vi "sub_SDR_siso_AWGN_channel.vi"(10 "Channel conf":T1, 11 "Shaped symbols":cdb[](array[numeric])) -> (3 "Array":cdb[](array[numeric]))   [LabVIEW 2012]
uses:
  <vilib>/Analysis/NI_AALBase.lvlib
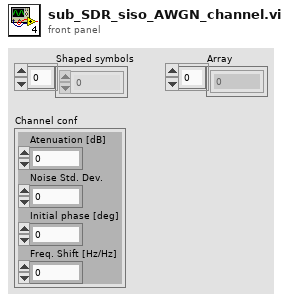
[diagram p1: front panel]
types:
  T1 = cluster{"Atenuation [dB]":dbl, "Noise Std. Dev.":dbl, "Initial phase [deg]":dbl, "Freq. Shift [Hz/Hz]":dbl}
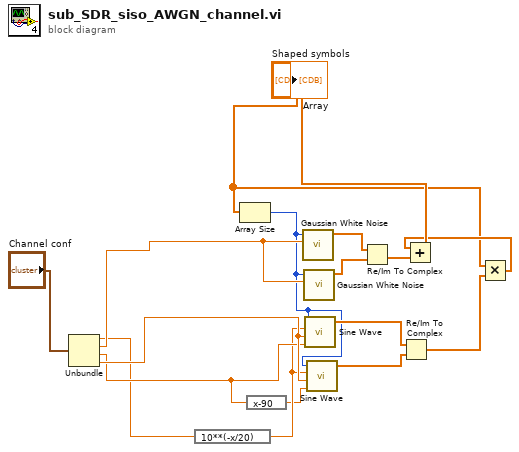
[diagram p0: block diagram]
diagram:
  n1 = Unbundle("Channel conf") -> ("Atenuation [dB]"=w14:dbl, "Noise Std. Dev."=w15:dbl, "Initial phase [deg]"=w16:dbl, "Freq. Shift [Hz/Hz]"=w17:dbl)
  n2 = expression code="10**(-x/20)"(w14) -> (w5:dbl)
  n3 = Array Size(array="Shaped symbols") -> (size(s)=w6:i32)
  n4 = expression code="x-90"(w16) -> (w4:dbl)
  n5 = call <vilib>:"Gaussian White Noise.vi"("standard deviation"=w15, "samples"=w6) -> ("Gaussian noise pattern"=w1:dbl[])  [unwired: 8 in, 1 out]
  n6 = call <vilib>:"Gaussian White Noise.vi"("standard deviation"=w15, "samples"=w6) -> ("Gaussian noise pattern"=w2:dbl[])  [unwired: 8 in, 1 out]
  n7 = call <vilib>:"Sine Wave.vi"("samples"=w6, "amplitude"=w5, "frequency"=w17, "phase in"=w16) -> ("sine wave"=w7:dbl[])  [unwired: 1 in, 2 out]
  n8 = call <vilib>:"Sine Wave.vi"("samples"=w6, "amplitude"=w5, "frequency"=w17, "phase in"=w4) -> ("sine wave"=w8:dbl[])  [unwired: 1 in, 2 out]
  n9 = Re/Im To Complex(1:w2, 2:w1) -> (0:w3:cdb[])
  n10 = Re/Im To Complex(1:w8, 2:w7) -> (0:w9:cdb[])
  n11 = Multiply(x="Shaped symbols", y=w9) -> (x*y=w11:cdb[])
  n12 = Add(x=w11, y=w3) -> (x+y=→"Array":cdb[])
